vi "Global stop.vi"() -> ()   [LabVIEW 2020]
panel:
  in  "Global stop":bool
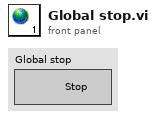
[diagram p1: front panel]
diagram:
